vi "Validate Hardware Custom Device.vi"(8 "error in (no error)":errorcluster, 11 "Hardware Ref in":T1 format="%.0x") -> (0 "error out":errorcluster, 3 "Hardware Ref out":T1 format="%.0x")   [LabVIEW 2020, in "Routing and Faulting Hardware API.lvlib"]
doc: "Asserts that the given Custom Device Ref is registered as a Routing and Faulting Hardware Custom Device and that the registered version is correct for this version of the API."
uses:
  Routing and Faulting Hardware API.lvlib
  <vilib>/NI VeriStand/Custom Device API/Custom Device Item Ref.ctl
  <vilib>/NI VeriStand/Custom Device API/Custom Device API.lvlib
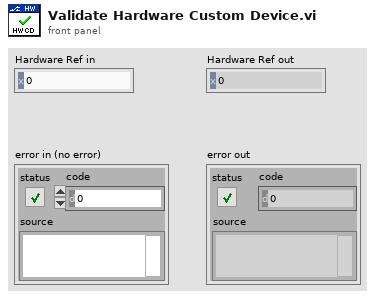
[diagram p1: front panel]
types:
  T1 = typedef "Custom Device API.lvlib/Custom Device Item Ref.ctl" = u64
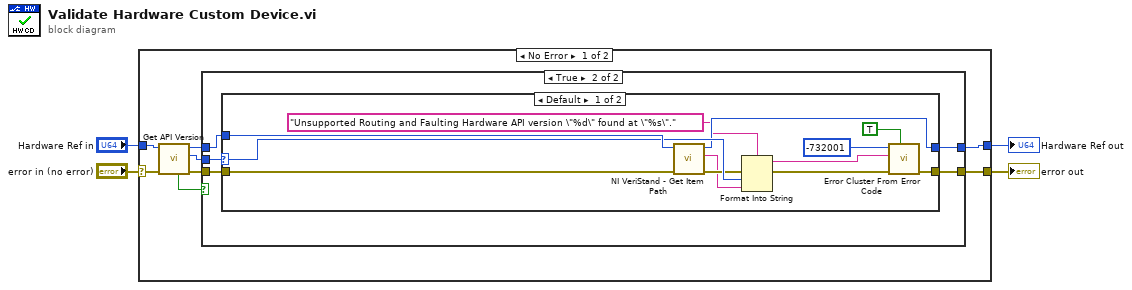
[diagram p0: block diagram]
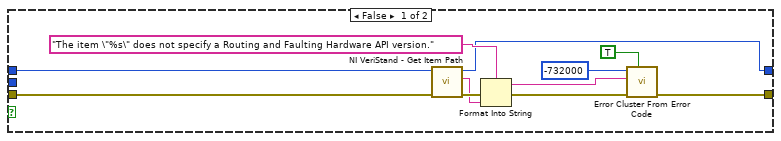
[diagram p2: hidden frame]
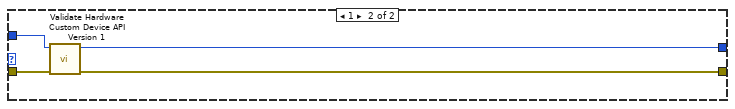
[diagram p3: hidden frame]
diagram:
  n1 = case shown="No Error" "error in (no error)" {
    selector: "error in (no error)" -> [w12 w46]
    tunnel: [w11 w46] -> w3
    tunnel: [w7 w45] -> w2
    tunnel: "Hardware Ref in" -> [w6 w45]
    frame No Error {
      n2 = call "Get API Version.vi"("error in (no error)"=w12, "Hardware Ref in"=w6) -> ("error out"=w10:errorcluster, "API version"=w8:u32, "Hardware Ref out"=w9:T1, "Found?"=w5:bool)  [unwired: 6 in]
      n3 = case shown="True" w5 {
        tunnel: [w16 w28] -> w11
        tunnel: w10 -> [w15 w27]
        tunnel: w9 -> [w14 w26]
        tunnel: w8 -> [_ w25]
        tunnel: [w13 w24] -> w7
        frame False {
          n4 = call <vilib>:"NI VeriStand - Get Item Path.vi"("error in (no error)"=w15, "Item Ref in"=w14) -> ("error out"=w22:errorcluster, "Path"=w20:string, "Item Ref out"=w13:T1)  [unwired: 6 in, 1 out]
          n5 = Format Into String(format string="The item \"%s\" does not specify a Routing and Faulting Hardware API version." ("error message (\"\")"), error in=w22, w20) -> (resulting string=w23:string, error out=w21:errorcluster)  [unwired: 1 in]
          n6 = call <vilib>:"Error Cluster From Error Code.vi"("show call chain? (False)"=TRUE, "error in (no error)"=w21, "error message (\"\")"=w23, "error code (0)"=-732000) -> ("error out"=w16:errorcluster)  [unwired: 5 in]
        }
        frame True {
          n7 = case shown="Default" w25 {
            selector: w25 -> [w37 _]
            tunnel: [w40 w43] -> w28
            tunnel: w27 -> [w39 w44]
            tunnel: w26 -> [w38 w41]
            tunnel: [w36 w42] -> w24
            frame Default {
              n8 = call <vilib>:"NI VeriStand - Get Item Path.vi"("error in (no error)"=w39, "Item Ref in"=w38) -> ("error out"=w34:errorcluster, "Path"=w32:string, "Item Ref out"=w36:T1)  [unwired: 6 in, 1 out]
              n9 = Format Into String(format string="Unsupported Routing and Faulting Hardware API version \"%d\" found at \"%s\"." ("error message (\"\")"), error in=w34, w37, w32) -> (resulting string=w35:string, error out=w33:errorcluster)  [unwired: 1 in]
              n10 = call <vilib>:"Error Cluster From Error Code.vi"("show call chain? (False)"=TRUE, "error in (no error)"=w33, "error message (\"\")"=w35, "error code (0)"=-732001) -> ("error out"=w40:errorcluster)  [unwired: 5 in]
            }
            frame 1 {
              n11 = call "Validate Hardware Custom Device API Version 1.vi"("error in (no error)"=w44, "Hardware Ref in"=w41) -> ("error out"=w43:errorcluster, "Hardware Ref out"=w42:T1)  [unwired: 8 in]
            }
          }
        }
      }
    }
    frame Error {
    }
  }
  "error out" <- w3
  "Hardware Ref out" <- w2
